vi "1D Time Stamp.vi"(5 "format string":string="%Y-%m-%dT%H:%M:%S%20u", 7 "key description":string, 8 "sections":string[](array[string]), 9 "time stamp":timestamp[](array[timestamp]), 11 "info data":string) -> (0 "sections out":string[](array[string]), 3 "info data out":string)   [LabVIEW 2013, in "infolib.lvlib"]
doc: "Add a new new date and time table to Info Data string. If section exists in Info Data string, inserts key into this section."
uses:
  infolib.lvlib
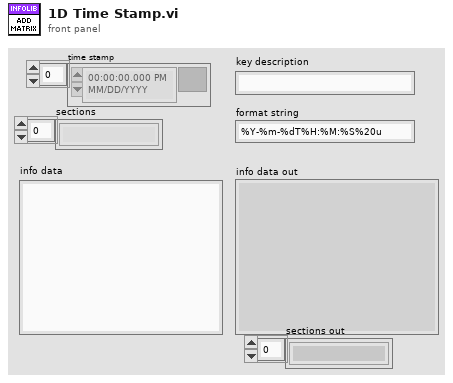
[diagram p1: front panel]
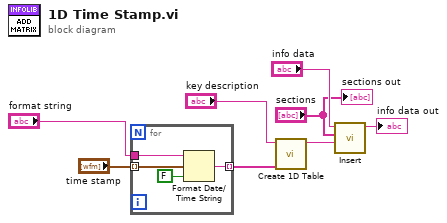
[diagram p0: block diagram]
diagram:
  n1 = for {
    tunnel: "format string" -> [w11]
    tunnel: "time stamp" -> [w12] mode=indexing
    tunnel: [w10] -> w3 mode=indexing
    n2 = Format Date/Time String(time format string (%c)=w11, seconds (now)=w12, UTC format=FALSE) -> (date/time string=w10:string)
  }
  n3 = call "Create 1D Table.vi"("formatted values"=w3, "table name"="key description") -> ("table"=w1:string)  [unwired: 9 in]
  n4 = call "Insert.vi"("insert"=w1, "sections"="sections", "info data"="info data") -> ("info data out"=→"info data out":string)  [unwired: 8 in]
  "sections out" <- "sections"
